vi "FTW-Setup.vi"() -> ()   [LabVIEW 2015]
panel:
  out "stderr":string
  out "stdout":string
  out "error out":errorcluster
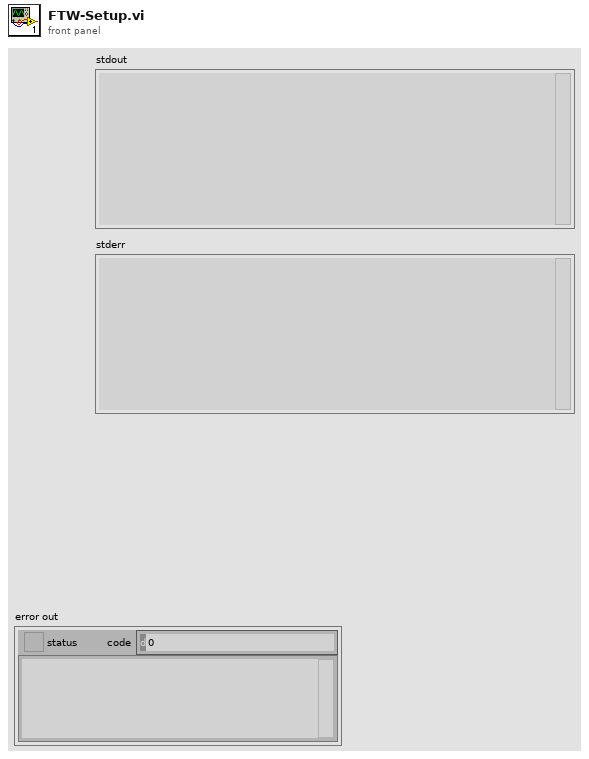
[diagram p1: front panel]
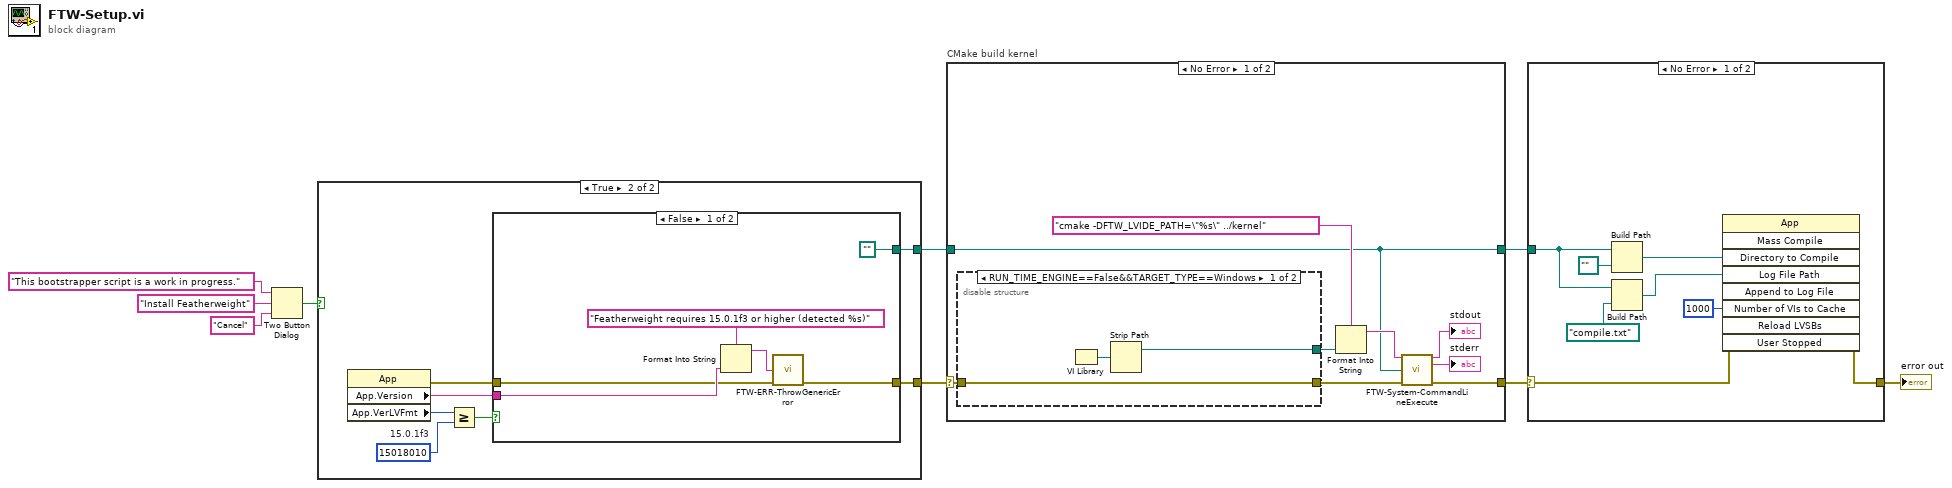
[diagram p0: block diagram]
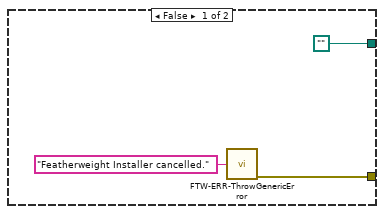
[diagram p2: hidden frame]
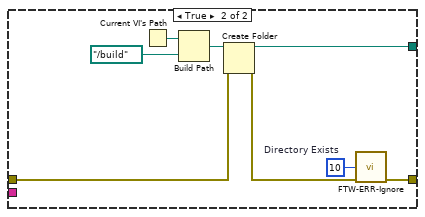
[diagram p3: hidden frame]
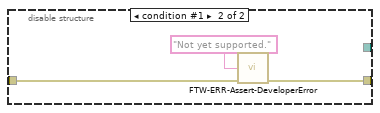
[diagram p4: hidden frame]
diagram:
  n1 = Two Button Dialog(message="This bootstrapper script is a work in progress.", 1:"Cancel" ("T button name (\"OK\")"), 2:"Install Featherweight" ("T button name (\"OK\")")) -> (T button?=w4:bool)
  n2 = case shown="True" w4 {
    tunnel: [w11 w15] -> w7
    tunnel: [path "" w13] -> w6
    frame False {
      n3 = call "FTW-ERR-ThrowGenericError.vi"("Error Message"="Featherweight Installer cancelled.") -> ("error out"=w11:errorcluster)  [unwired: 14 in]
    }
    frame True {
      w18 = 15018010  # 15.0.1f3
      n4 = property class="App"() -> (error out=w14:errorcluster, "App.Version"=w16:string, "App.VerLVFmt"=w19:i32)  [unwired: 2 in, 1 out]
      n5 = Greater Or Equal?(x=w19, y=w18) -> (x >= y?=w17:bool)
      n6 = case shown="False" w17 {
        tunnel: w16 -> [w24 _]
        tunnel: [w20 w26] -> w15
        tunnel: w14 -> [w21 w27]
        tunnel: [path "" w30] -> w13
        frame False {
          n7 = Format Into String(format string="Featherweight requires 15.0.1f3 or higher (detected %s)", w24) -> (resulting string=w22:string)  [unwired: 2 in, 1 out]
          n8 = call "FTW-ERR-ThrowGenericError.vi"("Error Message"=w22, "error in"=w21) -> ("error out"=w20:errorcluster)  [unwired: 13 in]
        }
        frame True {
          w29 = 10  # Directory Exists
          n9 = Current VI's Path() -> (path=w33:path)
          n10 = Build Path(base path=w33, name or relative path=path "../build" ("stripped path")) -> (appended path=w31:path)
          n11 = Create Folder(path (use dialog)=w31, error in=w27) -> (created path=w30:path, error out=w28:errorcluster)  [unwired: 1 in, 1 out]
          n12 = call "FTW-ERR-Ignore.vi"("Error Code"=w29, "error in"=w28) -> ("error out"=w26:errorcluster)  [unwired: 12 in, 1 out]
        }
      }
    }
  }
  n13 = case "CMake build kernel" shown="No Error" w7 {
    selector: w7 -> [w42 w50]
    tunnel: [w37 w50] -> w9
    tunnel: w6 -> [w36 w49]
    tunnel: [w36 w49] -> w3
    frame No Error {
      n14 = disable-structure shown="RUN_TIME_ENGINE==False&&TARGET_TYPE==Windows" {
        disable-tunnel: [w45 w47] -> w38
        disable-tunnel: w42 -> [w45 w48]
        disable-tunnel: [w44 _] -> w41
        frame condition #0 (active) {
          n15 = VI Library() -> (path=w43:path)
          n16 = Strip Path(path=w43) -> (stripped path=w44:path)  [unwired: 1 out]
        }
        frame condition #1 {
          n17 = call "FTW-ERR-Assert-DeveloperError.vi"("Reason this error should never happen"="Not yet supported.", "error in"=w48) -> ("error out"=w47:errorcluster)  [unwired: 13 in]
        }
      }
      n18 = Format Into String(format string="cmake -DFTW_LVIDE_PATH=\"%s\" ../kernel" ("command line"), w41) -> (resulting string=w39:string)  [unwired: 2 in, 1 out]
      n19 = call "FTW-System-CommandLineExecute.vi"("Command"=w39, "Working Directory"=w36, "error in"=w38) -> ("stdout"=→"stdout":string, "stderr"=→"stderr":string, "error out"=w37:errorcluster)  [unwired: 9 in, 1 out]
    }
    frame Error {
    }
  }
  n20 = case shown="No Error" w9 {
    selector: w9 -> [w55 w59]
    tunnel: [w54 w59] -> w8
    tunnel: w3 -> [w51 _]
    frame No Error {
      n21 = Build Path(base path=w51, name or relative path=path ".." ("stripped path")) -> (appended path=w52:path)
      n22 = Build Path(base path=w51, name or relative path=path "compile.txt" ("stripped path")) -> (appended path=w57:path)
      n23 = invoke class="App" method="Mass Compile"(error in=w55, "Directory to Compile"=w52, "Log File Path"=w57, "Number of VIs to Cache"=u32 1000) -> (error out=w54:errorcluster)  [unwired: 5 in, 8 out]
    }
    frame Error {
    }
  }
  "error out" <- w8
